vi "MDrive_Send_Parameters_File.vi"(3 "error in":errorcluster, 4 "parameters file":path=path "E:/thermionics/parameters.txt", 5 "VISA resource name in":refnum<visa-resource-name>) -> (0 "error in 2":errorcluster, 1 "Report":string, 2 "VISA resource name in 2":refnum<visa-resource-name>)   [LabVIEW 2017]
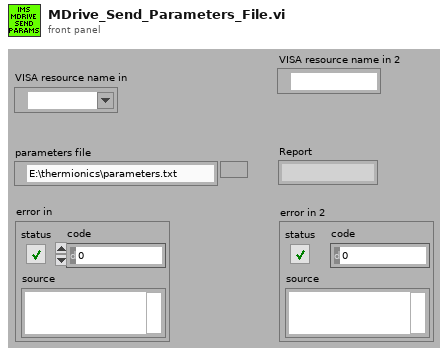
[diagram p1: front panel]
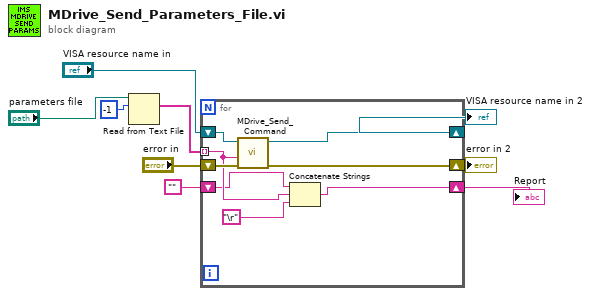
[diagram p0: block diagram]
diagram:
  n1 = Read from Text File(file (use dialog)="parameters file", count=-1) -> (text=w7:string[])  [unwired: 2 in, 3 out]
  n2 = for {
    shift-right: [w14] -> w5
    shift-left: "VISA resource name in" -> [w15]
    shift-right: [w16] -> w4
    shift-left: "error in" -> [w17]
    shift-right: [w12] -> w1
    shift-left: "" -> [w10]
    tunnel: w7 -> [w13] mode=indexing
    n3 = call "MDrive_Send_Command.vi"("error in"=w17, "Send String"=w13, "VISA resource name in"=w15) -> ("error out"=w16:errorcluster, "VISA resource name out"=w14:refnum<visa-resource-name>)  [unwired: 2 in, 1 out]
    n4 = Concatenate Strings(w10, w13, "\r") -> (w12:string)
  }
  "VISA resource name in 2" <- w5
  "error in 2" <- w4
  "Report" <- w1
